vi "HDI Bond Match.vi"(6 "Match Offset":cluster{"X":sgl, "Y":sgl}={"X"=133.0, "Y"=-3.0}, 8 "Minimum Match Score (Pattern Matching 1)":sgl=600.0, 9 "controller in":refnum<k24>, 10 "Template":path, 11 "Numeric":i32) -> (0 "error out":errorcluster, 1 "Number of Matches":i32, 3 "Match(es) Found":bool)   [LabVIEW 2011]
uses:
  C:/Users/Admin/Desktop/Gantry Code Transfer/source/Code Transfer/Aerotech.A3200.dll
  Aerotech.A3200.dll
  Template change for pattern match.vi
  <vilib>/vision/driver/NI_Vision_Acquisition_Software.lvlib
  <vilib>/vision/NI_Vision_Development_Module.lvlib
panel:
  in  "Scale Factor":sgl=0.000429
  out "y rel move":dbl
  out "x rel move":dbl
  out "y":sgl
  out "x":sgl
  out "Image Out":T1(plugin-control)
  out "Calibrated Matches":T2(array[cluster]) {"Bounding Box"."y" format="%.2f"; "Bounding Box"."x" format="%.2f"; "Position"."y" format="%.2f"; "Position"."x" format="%.2f"; "Score" format="%.2f"; "Scale" format="%.2f"; "Angle" format="%.2f"}
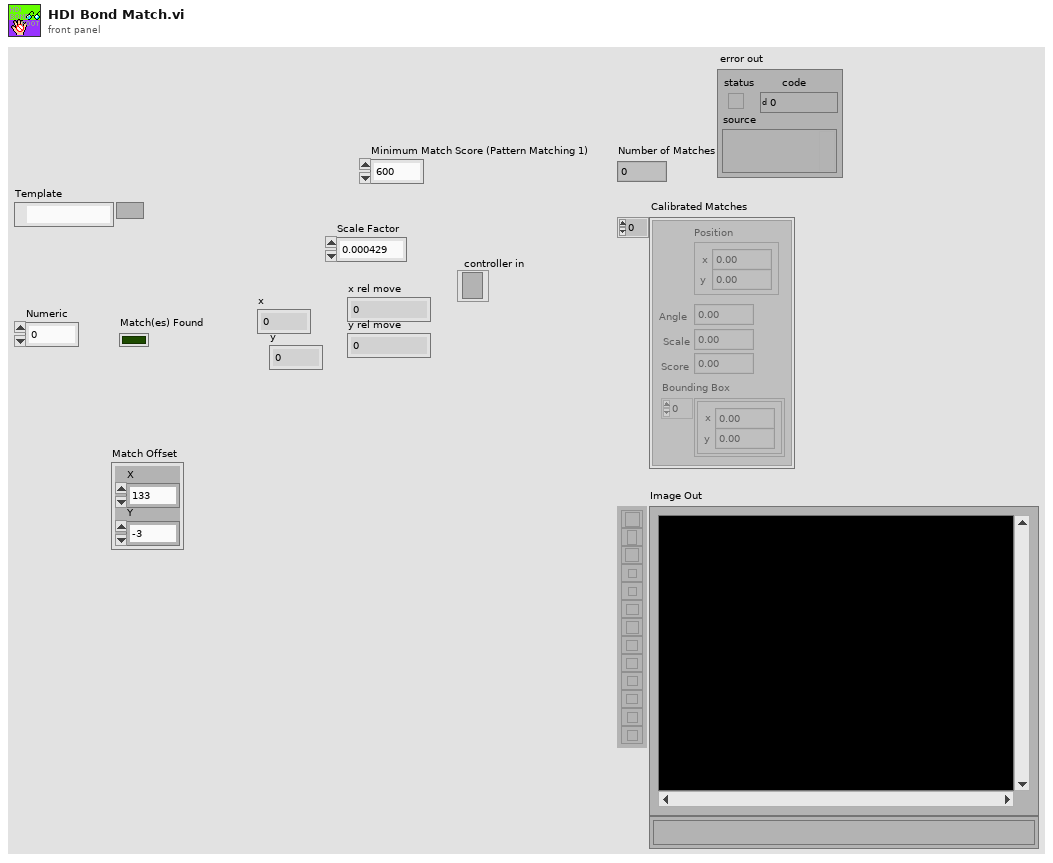
[diagram p1: front panel]
types:
  T1 = typedef "IMAQ Image.ctl" = refnum<image>
  T2 = cluster{"Position":cluster{"x":sgl, "y":sgl}, "Angle":sgl, "Scale":sgl, "Score":sgl, "Bounding Box":cluster{"x":sgl, "y":sgl}[]}[]
  T3 = cluster{"Global Rectangle":i32[], "Contours":cluster{"ID":enum32{"External", "Internal"}, "Type":u32, "Coordinates":i32[]}[]}
  T4 = typedef "IMAQdx.ctl" = refnum<k21>
  T5 = cluster{"Global Rectangle":i32[], "Number of Matches Requested":i32, "Minimum Match Score (Pattern Matching 1)":sgl}
  T6 = cluster{"Match Mode":u16, "Subpixel Accuracy":bool, "Rotation Angle Ranges (degrees)":cluster{sgl, sgl}[]}
  T7 = cluster{"Position":cluster{"x":sgl, "y":sgl}, "Angle":sgl, "Scale":sgl, "Score":sgl, "Bounding Box":cluster{"x":sgl, "y":sgl}[]}
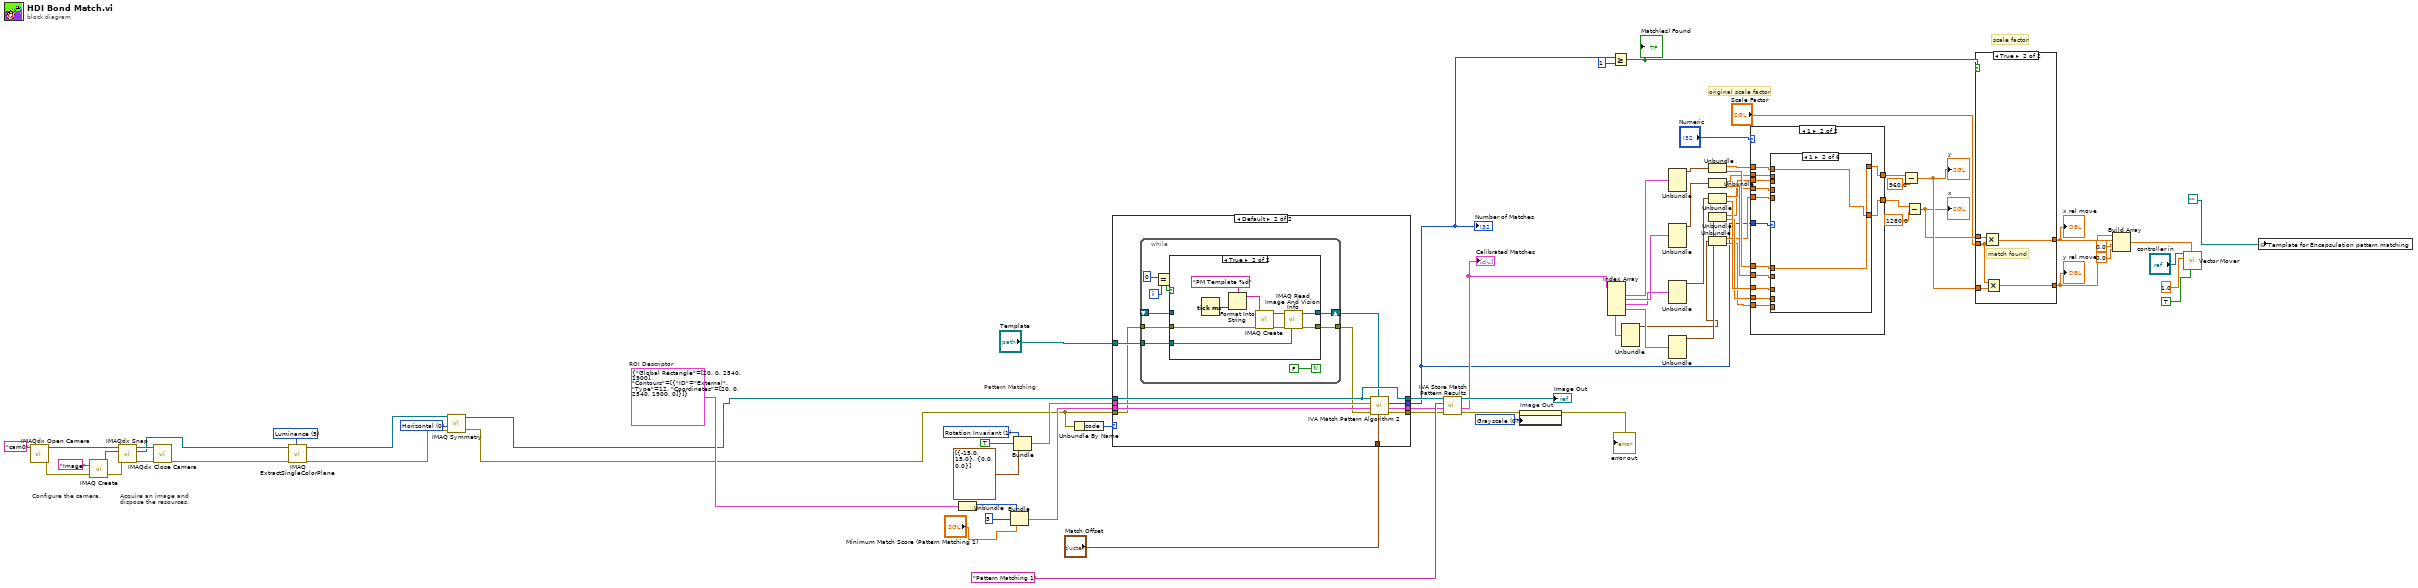
[diagram p0: block diagram]
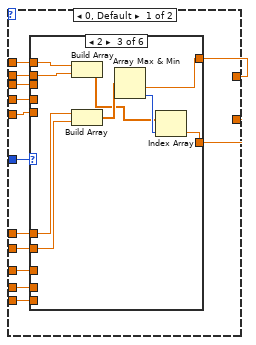
[diagram p2: hidden frame]
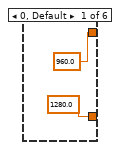
[diagram p3: hidden frame]
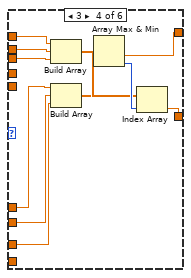
[diagram p5: hidden frame]
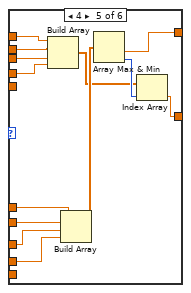
[diagram p6: hidden frame]
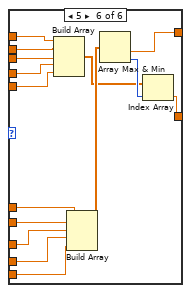
[diagram p7: hidden frame]
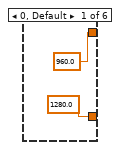
[diagram p8: hidden frame]
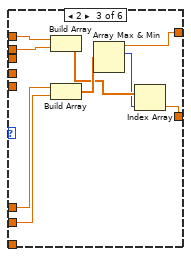
[diagram p9: hidden frame]
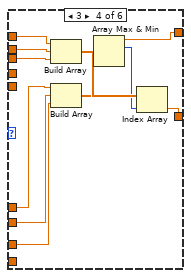
[diagram p10: hidden frame]
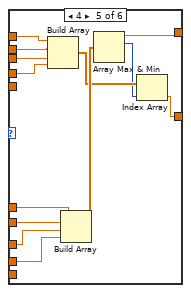
[diagram p11: hidden frame]
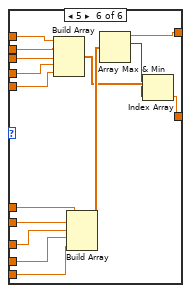
[diagram p12: hidden frame]
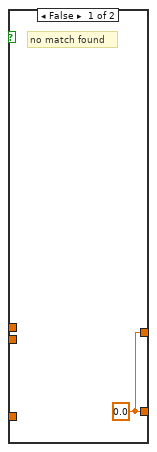
[diagram p13: hidden frame]
diagram:
  w5 = u32 0 items=["Horizontal", "Vertical", "Central", "1st Diagonal", "2nd Diagonal"] ("Type of Symmetry")
  w48 = u32 0 items=["Grayscale", "Binary", "Gradient", "Rainbow", "Temperature", "User Defined"] ("Palette")
  w65 = u16 1 items=["Shift Invariant", "Rotation Invariant"] ("Match Mode")
  w54 = T3 {"Global Rectangle"=[20, 0, 2540, 1900], "Contours"=[{"ID"=enum."External", "Type"=12, "Coordinates"=[20, 0, 2540, 1900, 0]}]}  # ROI Descriptor
  w67 = 5 items=["Red", "Green", "Blue", "Hue", "Saturation", "Luminance", "Value", "Intensity"] ("Color Plane")
  # "original scale factor"
  # "scale factor"
  # "Pattern Matching"
  # "Acquire an image and\ndispose the resources."
  # "Configure the camera."
  n1 = call <vilib>:"IMAQdx Open Camera.vi"("Session In"="cam0" ("Interface Name")) -> ("error out"=w74:errorcluster, "Session Out"=w68:T4)  [unwired: 9 in]
  n2 = call "IMAQ Create"("Image Name"="Image", "error in (no error)"=w74) -> ("New Image"=w70:T1, "error out"=w69:errorcluster)  [unwired: 3 in]
  n3 = call <vilib>:"IMAQdx Snap.vi"("error in"=w69, "Image In"=w70, "Session In"=w68) -> ("error out"=w72:errorcluster, "Image Out"=w66:T1, "Session Out"=w73:T4)  [unwired: 6 in]
  n4 = call <vilib>:"IMAQdx Close Camera.vi"("error in"=w72, "Session In"=w73) -> ("error out"=w71:errorcluster)  [unwired: 9 in]
  n5 = call "IMAQ ExtractSingleColorPlane"("Color Plane"=w67, "error in (no error)"=w71, "Image Src"=w66) -> ("error out"=w4:errorcluster, "Image Dst Out"=w3:T1)  [unwired: 7 in]
  n6 = call "IMAQ Symmetry"("error in (no error)"=w4, "Type of Symmetry"=w5, "Image Src"=w3) -> ("error out"=w1:errorcluster, "Image Dst Out"=w2:T1)  [unwired: 2 in]
  n7 = Unbundle(w54) -> ("Global Rectangle"=w53:i32[])  [unwired: 1 out]
  n8 = Bundle("Global Rectangle"=w53, "Number of Matches Requested"=5, "Minimum Match Score (Pattern Matching 1)"="Minimum Match Score (Pattern Matching 1)") -> (w59:T5)  [unwired: 1 in]
  n9 = Bundle("Match Mode"=w65, "Subpixel Accuracy"=TRUE, "Rotation Angle Ranges (degrees)"=cluster{sgl, sgl}[] [{-15.0, 15.0}, {0.0, 0.0}]) -> (w62:T6)  [unwired: 1 in]
  n10 = Unbundle By Name(w1) -> ("code"=w50:i32)
  n11 = case shown="Default" w50 {
    tunnel: "Template" -> [_ w81]
    tunnel: w1 -> [_ w80]
    tunnel: [_ w88] -> w11
    tunnel: w62 -> [_ w87]
    tunnel: w59 -> [_ w86]
    tunnel: "Match Offset" -> [_ w85]
    tunnel: w2 -> [w77 w82]
    tunnel: [_ w84] -> w56
    tunnel: [_ w83] -> w52
    tunnel: [w77 w82] -> w51
    frame -1074396199, -1074396198 {
      # "Discard\nCoordinate\nSystem Error"
    }
    frame Default {
      n12 = while {
        shift-right: [w97] -> w78
        shift-left: _ -> [w96]
        tunnel: [w94] -> w79
        tunnel: w80 -> [w93]
        tunnel: w81 -> [w92]
        i -> [w91]
        stop <- FALSE continue-if-true
        n13 = Equal?(x=0, y=w91) -> (x = y?=w89:bool)
        n14 = case shown="True" w89 {
          tunnel: [w99 w105] -> w97
          tunnel: w96 -> [w99 _]
          tunnel: [w98 w102] -> w94
          tunnel: w93 -> [w98 w101]
          tunnel: w92 -> [_ w100]
          frame False {
          }
          frame True {
            n15 = Tick Count (ms)() -> (millisecond timer value=w108:u32)
            n16 = Format Into String(format string="PM Template %d" ("Image Name"), w108) -> (resulting string=w107:string)  [unwired: 2 in, 1 out]
            n17 = call "IMAQ Create"("Image Name"=w107, "error in (no error)"=w101) -> ("New Image"=w104:T1, "error out"=w103:errorcluster)  [unwired: 3 in]
            n18 = call "IMAQ Read Image And Vision Info"("File Path"=w100, "error in (no error)"=w103, "Image"=w104) -> ("error out"=w102:errorcluster, "Image Out"=w105:T1)  [unwired: 6 in, 1 out]
          }
        }
      }
      n19 = call <vilib>:"IVA Match Pattern Algorithm 2.vi"("Match Offset"=w85, "Image Template"=w78, "error in (no error)"=w79, "Match Parameters"=w86, "Setup Match Parameters"=w87, "Image"=w82) -> ("error out"=w84:errorcluster, "Number of Matches"=w88:i32, "Matches"=w83:T2)  [unwired: 3 in]
    }
  }
  "Number of Matches" <- w11
  n20 = call <vilib>:"IVA Store Match Pattern Results.vi"("error in (no error)"=w56, "Matches"=w52, "Step Name"="Pattern Matching 1", "Image in"=w51) -> ("error out"=w55:errorcluster, "Calibrated Matches"=w13:T2, "Image dup"=→"Image Out":T1)  [unwired: 5 in]
  "Calibrated Matches" <- w13
  "error out" <- w55
  n21 = property on="Image Out" class="ImageControl"(error in=w55, "Palette:Palette Type"=w48) -> ()  [unwired: 1 in, 2 out]
  n22 = Index Array(array=w13) -> (element #1=w44:T7, element #2=w43:T7, element #3=w42:T7, element #4=w41:T7, element #5=w17:T7)  [unwired: 5 in]
  n23 = Greater Or Equal?(x=w11, y=1) -> (x >= y?=w31:bool)
  "Match(es) Found" <- w31
  n24 = Unbundle(w17) -> ("Position"=w16:cluster{"x":sgl, "y":sgl})  [unwired: 4 out]
  n25 = Unbundle(w44) -> ("Position"=w37:cluster{"x":sgl, "y":sgl})  [unwired: 4 out]
  n26 = Unbundle(w43) -> ("Position"=w38:cluster{"x":sgl, "y":sgl})  [unwired: 4 out]
  n27 = Unbundle(w42) -> ("Position"=w39:cluster{"x":sgl, "y":sgl})  [unwired: 4 out]
  n28 = Unbundle(w41) -> ("Position"=w40:cluster{"x":sgl, "y":sgl})  [unwired: 4 out]
  n29 = Unbundle(w37) -> ("x"=w27:sgl, "y"=w26:sgl)
  n30 = Unbundle(w38) -> ("x"=w25:sgl, "y"=w24:sgl)
  n31 = Unbundle(w39) -> ("x"=w22:sgl, "y"=w21:sgl)
  n32 = Unbundle(w40) -> ("x"=w18:sgl, "y"=w20:sgl)
  n33 = Unbundle(w16) -> ("x"=w15:sgl, "y"=w14:sgl)
  n34 = case shown="1" "Numeric" {
    tunnel: w27 -> [w121 w186]
    tunnel: w26 -> [w120 w181]
    tunnel: w25 -> [w119 w185]
    tunnel: w24 -> [w118 w180]
    tunnel: [w117 w174] -> w23
    tunnel: w22 -> [w116 w184]
    tunnel: w21 -> [w115 w179]
    tunnel: w20 -> [w114 w178]
    tunnel: [w113 w175] -> w19
    tunnel: w18 -> [w112 w183]
    tunnel: w15 -> [w111 w182]
    tunnel: w14 -> [w110 w177]
    tunnel: w11 -> [w109 w176]
    frame 0, Default {
      n35 = case shown="2" w109 {
        tunnel: w121 -> [_ w124 w134 w142 w155 w170]
        tunnel: w120 -> [_ w125 w132 w139 w151 w166]
        tunnel: [sgl 960.0 ("y") w125 w129 w144 w157 w172] -> w117
        tunnel: w119 -> [_ _ w133 w141 w154 w169]
        tunnel: w118 -> [_ _ w131 w138 w150 w165]
        tunnel: w116 -> [_ _ _ w140 w153 w168]
        tunnel: w115 -> [_ _ _ w137 w149 w164]
        tunnel: w114 -> [_ _ _ _ w148 w163]
        tunnel: [sgl 1280.0 ("x") w124 w126 w143 w156 w171] -> w113
        tunnel: w112 -> [_ _ _ _ w152 w167]
        tunnel: w111 -> [_ _ _ _ _ w160]
        tunnel: w110 -> [_ _ _ _ _ w159]
        frame 0, Default {
        }
        frame 1 {
        }
        frame 2 {
          n36 = Build Array(w134, w133) -> (w127:sgl[])
          n37 = Build Array(w132, w131) -> (w128:sgl[])
          n38 = Array Max & Min(array=w128) -> (min value=w129:sgl, min index (indices)=w130:i32)  [unwired: 2 out]
          n39 = Index Array(array=w127, index=w130) -> (element=w126:sgl)
        }
        frame 3 {
          n40 = Build Array(w142, w141, w140) -> (w136:sgl[])
          n41 = Build Array(w139, w138, w137) -> (w135:sgl[])
          n42 = Array Max & Min(array=w135) -> (min value=w144:sgl, min index (indices)=w145:i32)  [unwired: 2 out]
          n43 = Index Array(array=w136, index=w145) -> (element=w143:sgl)
        }
        frame 4 {
          n44 = Build Array(w155, w154, w153, w152) -> (w146:sgl[])
          n45 = Build Array(w151, w150, w149, w148) -> (w147:sgl[])
          n46 = Array Max & Min(array=w147) -> (min value=w157:sgl, min index (indices)=w158:i32)  [unwired: 2 out]
          n47 = Index Array(array=w146, index=w158) -> (element=w156:sgl)
        }
        frame 5 {
          n48 = Build Array(w170, w169, w168, w167, w160) -> (w161:sgl[])
          n49 = Build Array(w166, w165, w164, w163, w159) -> (w162:sgl[])
          n50 = Array Max & Min(array=w162) -> (min value=w172:sgl, min index (indices)=w173:i32)  [unwired: 2 out]
          n51 = Index Array(array=w161, index=w173) -> (element=w171:sgl)
        }
      }
    }
    frame 1 {
      n52 = case shown="1" w176 {
        tunnel: w186 -> [_ w189 w199 w209 w222 w237]
        tunnel: w181 -> [_ w190 w197 w206 w218 w233]
        tunnel: [sgl 960.0 ("y") w190 w192 w201 w212 w225] -> w174
        tunnel: w185 -> [_ _ w198 w208 w221 w236]
        tunnel: w180 -> [_ _ w196 w205 w217 w232]
        tunnel: w184 -> [_ _ _ w207 w220 w235]
        tunnel: w179 -> [_ _ _ w204 w216 w231]
        tunnel: w178 -> [_ _ _ _ w215 w230]
        tunnel: [sgl 1280.0 ("x") w189 w193 w210 w223 w238] -> w175
        tunnel: w183 -> [_ _ _ _ w219 w234]
        tunnel: w182 -> [_ _ _ _ _ w227]
        tunnel: w177 -> [_ _ _ _ _ w226]
        frame 0, Default {
        }
        frame 1 {
        }
        frame 2 {
          n53 = Build Array(w199, w198) -> (w194:sgl[])
          n54 = Build Array(w197, w196) -> (w195:sgl[])
          n55 = Array Max & Min(array=w195) -> (max value=w192:sgl, max index (indices)=w191:i32)  [unwired: 2 out]
          n56 = Index Array(array=w194, index=w191) -> (element=w193:sgl)
        }
        frame 3 {
          n57 = Build Array(w209, w208, w207) -> (w203:sgl[])
          n58 = Build Array(w206, w205, w204) -> (w202:sgl[])
          n59 = Array Max & Min(array=w202) -> (max value=w201:sgl, max index (indices)=w200:i32)  [unwired: 2 out]
          n60 = Index Array(array=w203, index=w200) -> (element=w210:sgl)
        }
        frame 4 {
          n61 = Build Array(w222, w221, w220, w219) -> (w213:sgl[])
          n62 = Build Array(w218, w217, w216, w215) -> (w214:sgl[])
          n63 = Array Max & Min(array=w214) -> (max value=w212:sgl, max index (indices)=w211:i32)  [unwired: 2 out]
          n64 = Index Array(array=w213, index=w211) -> (element=w223:sgl)
        }
        frame 5 {
          n65 = Build Array(w237, w236, w235, w234, w227) -> (w228:sgl[])
          n66 = Build Array(w233, w232, w231, w230, w226) -> (w229:sgl[])
          n67 = Array Max & Min(array=w229) -> (max value=w225:sgl, max index (indices)=w224:i32)  [unwired: 2 out]
          n68 = Index Array(array=w228, index=w224) -> (element=w238:sgl)
        }
      }
    }
  }
  n69 = Subtract(x=w23, y=sgl 960.0) -> (x-y=w47:sgl)
  "y" <- w47
  n70 = Subtract(x=w19, y=sgl 1280.0) -> (x-y=w46:sgl)
  "x" <- w46
  n71 = case shown="True" w31 {
    tunnel: w47 -> [_ w244]
    tunnel: w46 -> [_ w243]
    tunnel: [w239 w242] -> w29
    tunnel: [w239 w241] -> w30
    tunnel: "Scale Factor" -> [_ w240]
    frame False {
      w239 = sgl 0.0
      # "no match found"
    }
    frame True {
      # "match found"
      n72 = Multiply(x=w243, y=w240) -> (x*y=w242:sgl)
      n73 = Multiply(x=w240, y=w244) -> (x*y=w241:sgl)
    }
  }
  "x rel move" <- w29
  "y rel move" <- w30
  n74 = Build Array(w30, w29, 0.0 ("element"), 0.0 ("element")) -> (w32:dbl[])
  n75 = call "Vector Mover.vi"("Absolute/Relative (F/T)"=TRUE, "Movement Vector"=w32, "Vector Speed"=1.0, "controller in"="controller in") -> ()  [unwired: 2 in, 4 out]
  n76 = global write "Template change for pattern match.vi" "Template for Encapsulation pattern matching"(path "") -> ()
